vi "histogram.vi"(6 "Percentile check":dbl, 7 "Image ROI":T1, 8 "useROI":bool, 9 "ROI Descriptor":T3 {"Contours"."Type" items=["No Selection", "Point", "Line", "Rectangle", "Oval", "Polygon", "Freehand Region", "Annulus", "Unused2", "Unused3", "Broken Line", "Freehand Line", "Rotated Rectangle"]}, 10 "bit depth":enum16{"16bits", "14bits", "12bits", "8bits"}(ring), 11 "Image":T1) -> (0 "error out":errorcluster, 1 "Statistics":T2 {"# Sat. Pixels" scale=0.0..10.0}, 2 "Histograph":T4(graph)={"Starting Value"=-32768.0, "Incremental Value"=1.0, "Histogram"=array[65536 elements]}, 3 "Image Out (ROI)":T1, 4 "bins":i32)   [LabVIEW 2023]
uses:
  <vilib>/vision/Image Controls.llb/IMAQ Image.ctl
  <vilib>/vision/NI_Vision_Development_Module.lvlib
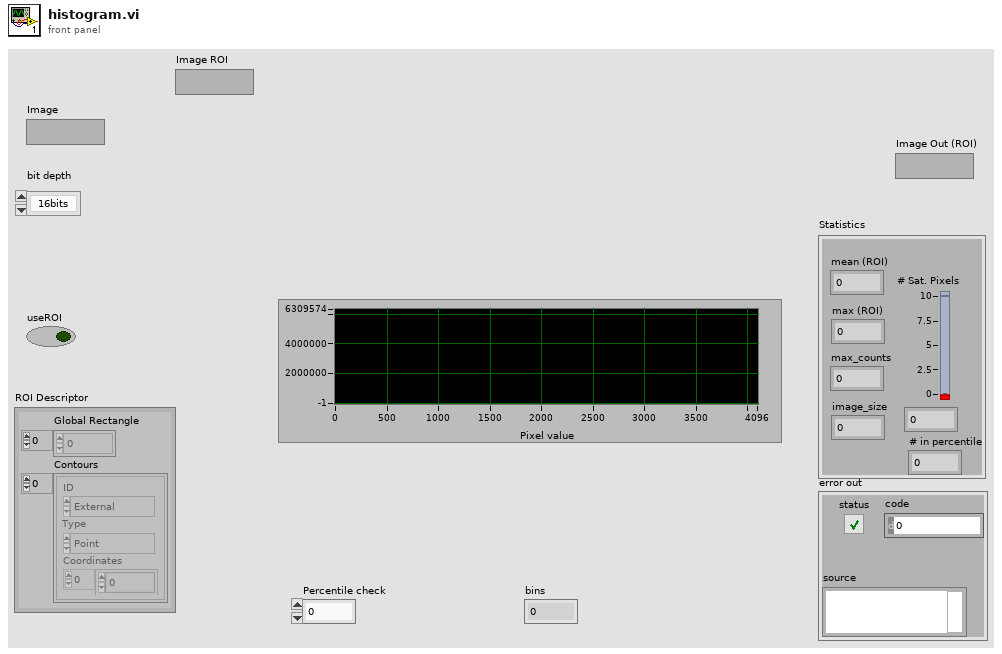
[diagram p1: front panel]
types:
  T1 = typedef "IMAQ Image.ctl" = refnum<image>
  T2 = cluster{"mean (ROI)":dbl, "max (ROI)":i16, "max_counts":dbl, "image_size":i32, "# Sat. Pixels":sgl, "# in percentile":dbl}
  T3 = cluster{"Global Rectangle":i32[], "Contours":cluster{"ID":enum32{"External", "Internal"}, "Type":u32, "Coordinates":i32[]}[]}
  T4 = cluster{"Starting Value":sgl, "Incremental Value":sgl, "Histogram":u32[]}
  T5 = cluster{"ID":enum32{"External", "Internal"}, "Type":u32, "Coordinates":i32[]}[]
  T6 = cluster{"ID":enum32{"External", "Internal"}, "Type":u32, "Coordinates":i32[]}
  T7 = cluster{"mean":dbl, u16, sgl, "size":i32, u32, u32}
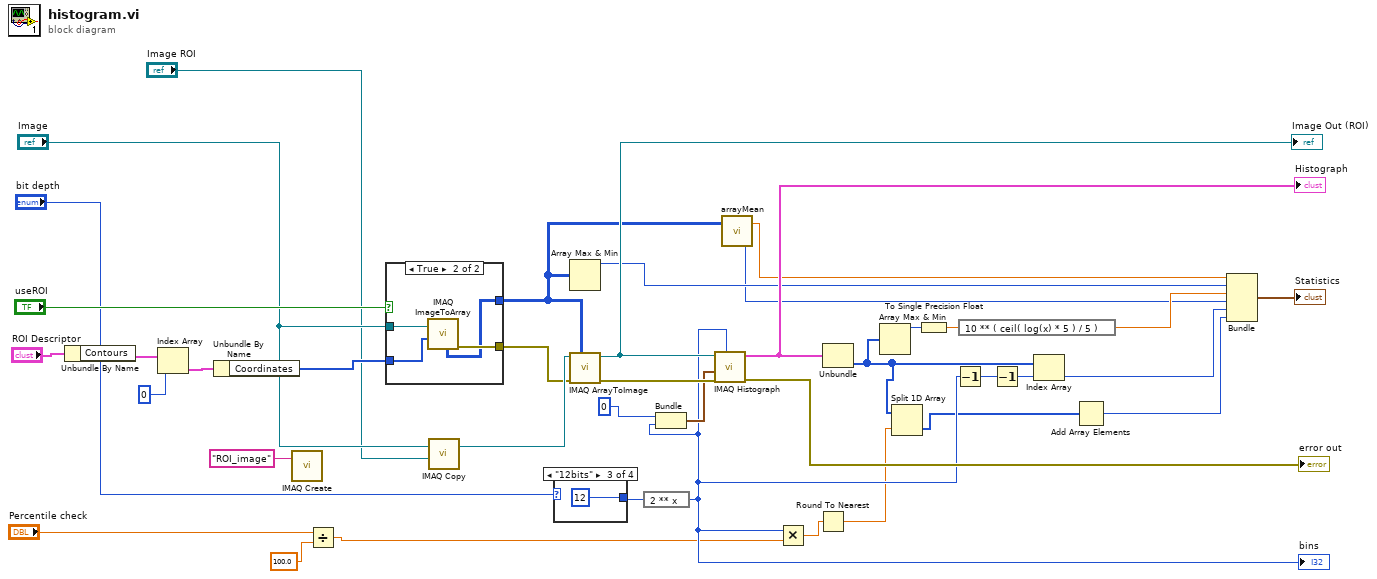
[diagram p0: block diagram]
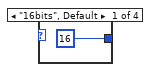
[diagram p2: hidden frame]
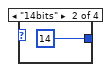
[diagram p3: hidden frame]
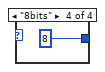
[diagram p4: hidden frame]
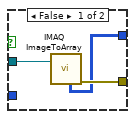
[diagram p5: hidden frame]
diagram:
  n1 = Unbundle By Name("ROI Descriptor") -> ("Contours"=w22:T5)
  n2 = Index Array(array=w22, index=0) -> (element=w17:T6)
  n3 = Unbundle By Name(w17) -> ("Coordinates"=w20:i32[])
  n4 = call "IMAQ Create"("Image Name"="ROI_image") -> ()  [unwired: 4 in, 2 out]
  n5 = Divide(x="Percentile check", y=100.0) -> (x/y=w8:dbl)
  n6 = case shown="True" "useROI" {
    tunnel: [w40 w44] -> w16
    tunnel: "Image" -> [w41 w46]
    tunnel: [w42 w45] -> w25
    tunnel: w20 -> [_ w43]
    frame False {
      n7 = call "IMAQ ImageToArray"("Image"=w41) -> ("Image Pixels (U16)"=w40:u16[][], "error out"=w42:errorcluster)  [unwired: 3 in, 3 out]
    }
    frame True {
      n8 = call "IMAQ ImageToArray"("Optional Rectangle"=w43, "Image"=w46) -> ("Image Pixels (U16)"=w44:u16[][], "error out"=w45:errorcluster)  [unwired: 2 in, 3 out]
    }
  }
  n9 = call "IMAQ Copy"("Image Dst"="Image ROI", "Image Src"="Image") -> ("Image Dst Out"=w32:T1)  [unwired: 4 in, 1 out]
  n10 = case shown="\"12bits\"" "bit depth" {
    tunnel: [16 14 12 8] -> w26
    frame "16bits", Default {
    }
    frame "14bits" {
    }
    frame "12bits" {
    }
    frame "8bits" {
    }
  }
  n11 = Array Max & Min(array=w16) -> (max value=w29:u16)  [unwired: 3 out]
  n12 = call "IMAQ ArrayToImage"("Image Pixels (U16)"=w16, "error in (no error)"=w25, "Image"=w32) -> ("error out"=w24:errorcluster, "Image Out"=w34:T1)  [unwired: 7 in]
  "Image Out (ROI)" <- w34
  n13 = expression code="2 ** x"(w26) -> (w10:i32)
  "bins" <- w10
  n14 = Bundle(0, w10) -> (w18:cluster{i32, i32})  [unwired: 1 in]
  n15 = call "IMAQ Histograph"("Number of Classes"=w10, "error in (no error)"=w24, "Interval Range"=w18, "Image"=w34) -> ("error out"=→"error out":errorcluster, "Histogram Graph"=w39:T4)  [unwired: 4 in, 2 out]
  "Histograph" <- w39
  n16 = call "arrayMean.vi"("Array"=w16) -> ("size"=w14:i32, "mean"=w15:dbl)  [unwired: 1 in]
  n17 = Multiply(x=w10, y=w8) -> (x*y=w7:dbl)
  n18 = Round To Nearest(number=w7) -> (nearest integer value=w3:dbl)
  n19 = Unbundle(w39) -> ("Histogram"=w4:u32[])  [unwired: 2 out]
  n20 = Array Max & Min(array=w4) -> (max value=w31:u32)  [unwired: 3 out]
  n21 = Split 1D Array(array=w4, index=w3) -> (second subarray=w2:u32[])  [unwired: 1 out]
  n22 = To Single Precision Float(number=w31) -> (single precision float=w30:sgl)
  n23 = Decrement(x=w10) -> (x-1=w12:i32)
  n24 = expression code="10 ** ( ceil( log(x) * 5 ) / 5 )"(w30) -> (w23:sgl)
  n25 = Decrement(x=w12) -> (x-1=w11:i32)
  n26 = Index Array(array=w4, index=w11) -> (element=w28:u32)
  n27 = Add Array Elements(numeric array=w2) -> (sum=w1:u32)
  n28 = Bundle("mean"=w15, w29, w23, "size"=w14, w28, w1) -> (→"Statistics":T7)  [unwired: 1 in]
